vi "Setting.vi"() -> ()   [LabVIEW 2020]
uses:
  <userlib>/_MGI/1D Array/MGI Average/MGI Average (DBL[]).vi
  Global_Variable/Global.vi
  Libraries/S7/S7.lvlib
panel:
  in  "停止":bool
  in  "输入轴标定":bool
  out "标定曲线":cluster{dbl[], dbl[]}[](graph)
  # "配置标定"
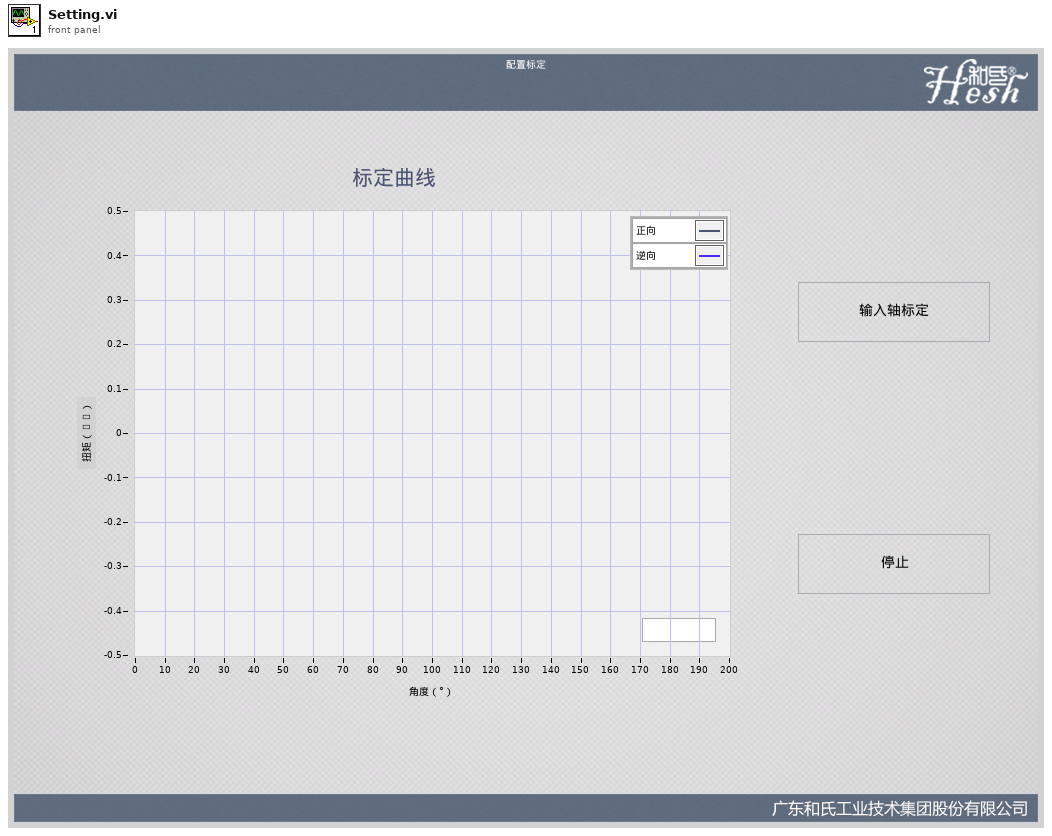
[diagram p1: front panel]
types:
  T1 = cluster{"输入旋转位移":sgl, "位移":sgl, "工装移载位移":sgl, "输入编码位移":sgl, "输入扭矩":sgl, "输出扭矩(小)":sgl, "拉压力":sgl, "吸收电流":sgl}
  T2 = cluster{"输入轴扭矩":dbl, "输出轴扭矩小量程":dbl, "输出轴扭矩大量程":dbl}
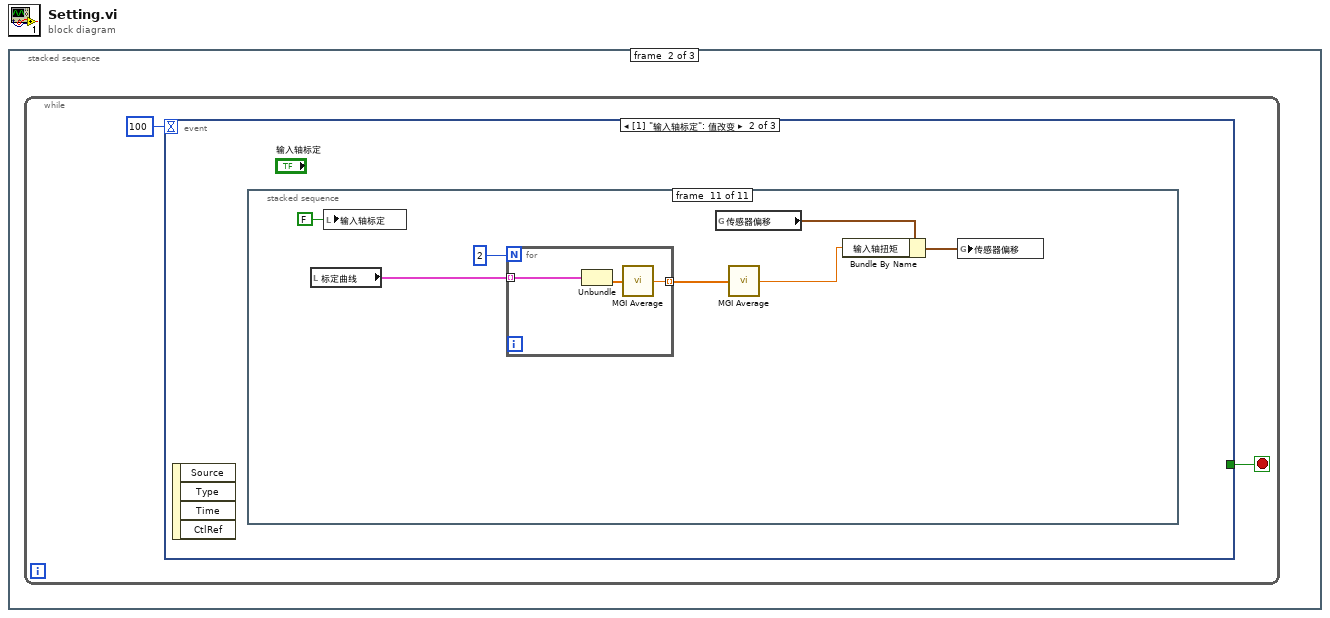
[diagram p0: block diagram]
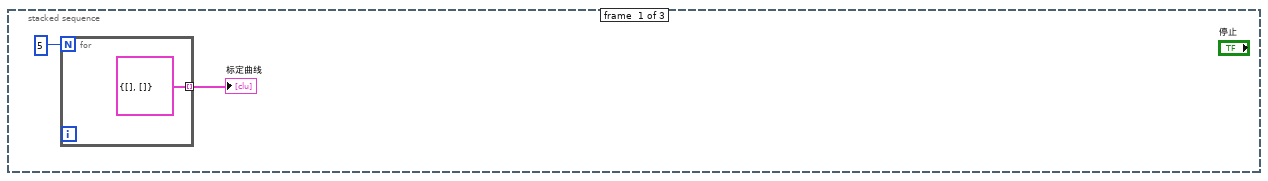
[diagram p2: hidden frame]
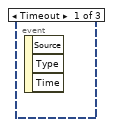
[diagram p3: hidden frame]
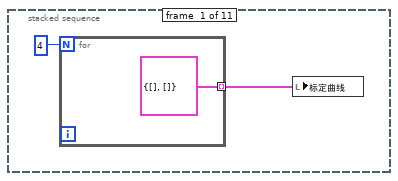
[diagram p4: hidden frame]
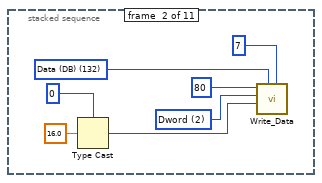
[diagram p5: hidden frame]
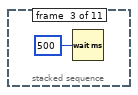
[diagram p6: hidden frame]
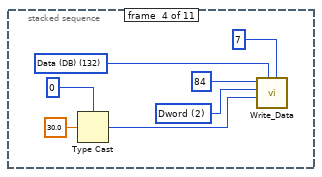
[diagram p7: hidden frame]
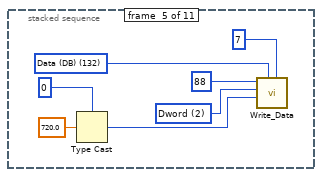
[diagram p8: hidden frame]
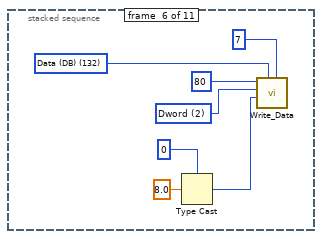
[diagram p9: hidden frame]
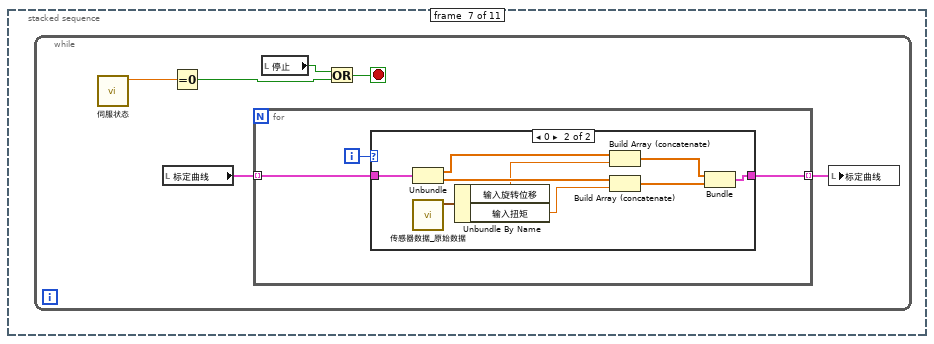
[diagram p10: hidden frame]
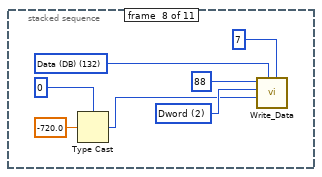
[diagram p12: hidden frame]
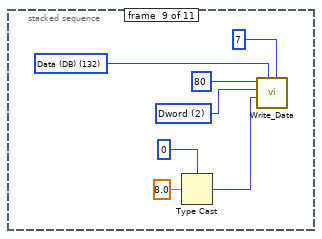
[diagram p13: hidden frame]
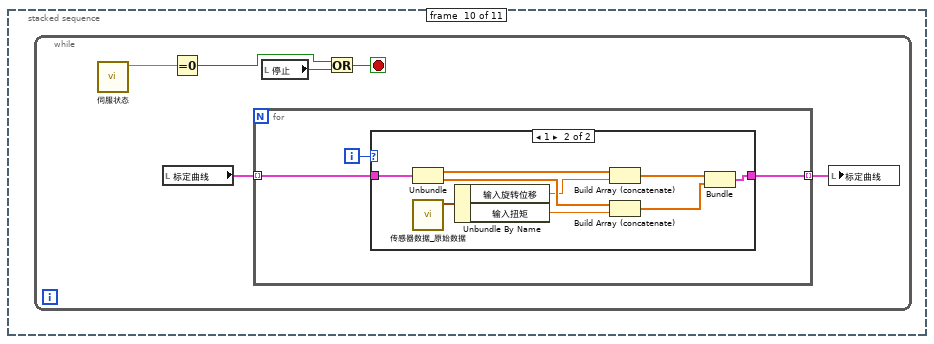
[diagram p14: hidden frame]
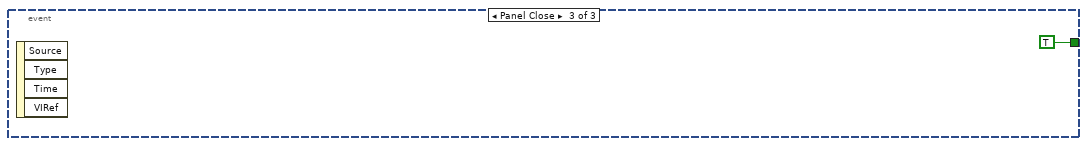
[diagram p16: hidden frame]
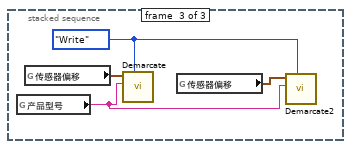
[diagram p17: hidden frame]
diagram:
  n1 = stacked-sequence {
    frame #0 {
      n2 = for {
        N: 5 -> [_]
        tunnel: [cluster{dbl[], dbl[]} {[], []}] -> w1 mode=indexing
      }
      "标定曲线" <- w1
    }
    frame #1 {
      n3 = while {
        stop <- w5 stop-if-true
        n4 = event shown="[1] \"输入轴标定\": 值改变" {
          selector: _ -> [_ _ _]
          dyn-events: _ -> [_ _ _]
          timeout: 100 -> [_ _ _]
          tunnel: [_ _ TRUE] -> w5
          event Timeout {
            n5 = event-data() -> ()  [unwired: 1 in, 3 out]
          }
          event "输入轴标定": Value Change {
            n6 = event-data() -> ()  [unwired: 1 in, 4 out]
            n7 = stacked-sequence {
              frame #0 {
                n8 = for {
                  N: 4 -> [_]
                  tunnel: [cluster{dbl[], dbl[]} {[], []}] -> w7 mode=indexing
                }
                n9 = local write "标定曲线"(w7) -> ()
              }
              frame #1 {
                w13 = u16 2 items=["byte", "word", "Dword"] ("数据类型")
                w15 = u8 132 items=["I/O (P)"=128, "Input (I)"=129, "Output (Q)"=130, "Bit Memory (M)"=131, "Data (DB)"=132, "Instance Data (DI)"=133, "Local Data (L)"=134, "Predecessor Local Data (VL)"=135] ("寄存器类型")
                n10 = Type Cast(type=u32 0, x=sgl 16.0 ("输入轴旋转绝对位置")) -> (*(type *) &x=w11:u32)
                n11 = call "Write_Data.vi"("DB #"=u16 7, "寄存器类型"=w15, "写入数据"=w11, "数据类型"=w13, "写入地址"=u32 80) -> ()  [unwired: 4 in, 3 out]
              }
              frame #2 {
                n12 = Wait (ms)(milliseconds to wait=u32 500 ("等待时间（毫秒）")) -> ()  [unwired: 1 out]
              }
              frame #3 {
                w21 = u16 2 items=["byte", "word", "Dword"] ("数据类型")
                w23 = u8 132 items=["I/O (P)"=128, "Input (I)"=129, "Output (Q)"=130, "Bit Memory (M)"=131, "Data (DB)"=132, "Instance Data (DI)"=133, "Local Data (L)"=134, "Predecessor Local Data (VL)"=135] ("寄存器类型")
                n13 = Type Cast(type=u32 0, x=sgl 30.0 ("输入轴旋转绝对位置")) -> (*(type *) &x=w19:u32)
                n14 = call "Write_Data.vi"("DB #"=u16 7, "寄存器类型"=w23, "写入数据"=w19, "数据类型"=w21, "写入地址"=u32 84) -> ()  [unwired: 4 in, 3 out]
              }
              frame #4 {
                w27 = u16 2 items=["byte", "word", "Dword"] ("数据类型")
                w28 = u8 132 items=["I/O (P)"=128, "Input (I)"=129, "Output (Q)"=130, "Bit Memory (M)"=131, "Data (DB)"=132, "Instance Data (DI)"=133, "Local Data (L)"=134, "Predecessor Local Data (VL)"=135] ("寄存器类型")
                n15 = Type Cast(type=u32 0, x=sgl 720.0 ("输入轴旋转绝对位置")) -> (*(type *) &x=w30:u32)
                n16 = call "Write_Data.vi"("DB #"=u16 7, "寄存器类型"=w28, "写入数据"=w30, "数据类型"=w27, "写入地址"=u32 88) -> ()  [unwired: 4 in, 3 out]
              }
              frame #5 {
                w34 = u16 2 items=["byte", "word", "Dword"] ("数据类型")
                w35 = u8 132 items=["I/O (P)"=128, "Input (I)"=129, "Output (Q)"=130, "Bit Memory (M)"=131, "Data (DB)"=132, "Instance Data (DI)"=133, "Local Data (L)"=134, "Predecessor Local Data (VL)"=135] ("寄存器类型")
                n17 = Type Cast(type=u32 0, x=sgl 8.0 ("输入轴旋转绝对位置")) -> (*(type *) &x=w37:u32)
                n18 = call "Write_Data.vi"("DB #"=u16 7, "寄存器类型"=w35, "写入数据"=w37, "数据类型"=w34, "写入地址"=u32 80) -> ()  [unwired: 4 in, 3 out]
              }
              frame #6 {
                n19 = while {
                  stop <- w42 stop-if-true
                  n20 = call "伺服状态.vi"() -> ("Status"=w39:sgl)  [unwired: 11 in]
                  n21 = local read "标定曲线"() -> (w41:cluster{dbl[], dbl[]}[])
                  n22 = Equal To 0?(x=w39) -> (x = 0?=w38:bool)
                  n23 = for {
                    tunnel: [w44] -> w40 mode=indexing
                    tunnel: w41 -> [w46] mode=indexing
                    i -> [w45]
                    n24 = case shown="0" w45 {
                      tunnel: [w47 w51] -> w44
                      tunnel: w46 -> [w47 w52]
                      frame Default {
                      }
                      frame 0 {
                        n25 = Unbundle(w52) -> (w56:dbl[], w55:dbl[])
                        n26 = call "传感器数据_原始数据.vi"() -> ("传感器读数"=w50:T1)  [unwired: 11 in]
                        n27 = Unbundle By Name(w50) -> ("输入旋转位移"=w49:sgl, "输入扭矩"=w48:sgl)
                        n28 = Build Array (concatenate)(w56, w49) -> (w54:dbl[])
                        n29 = Build Array (concatenate)(w55, w48) -> (w53:dbl[])
                        n30 = Bundle(w54, w53) -> (w51:cluster{dbl[], dbl[]})  [unwired: 1 in]
                      }
                    }
                  }
                  n31 = local read "停止"() -> (w43:bool)
                  n32 = Or(x=w43, y=w38) -> (x .or. y?=w42:bool)
                  n33 = local write "标定曲线"(w40) -> ()
                }
              }
              frame #7 {
                w61 = u16 2 items=["byte", "word", "Dword"] ("数据类型")
                w63 = u8 132 items=["I/O (P)"=128, "Input (I)"=129, "Output (Q)"=130, "Bit Memory (M)"=131, "Data (DB)"=132, "Instance Data (DI)"=133, "Local Data (L)"=134, "Predecessor Local Data (VL)"=135] ("寄存器类型")
                n34 = Type Cast(type=u32 0, x=sgl -720.0 ("输入轴旋转绝对位置")) -> (*(type *) &x=w59:u32)
                n35 = call "Write_Data.vi"("DB #"=u16 7, "寄存器类型"=w63, "写入数据"=w59, "数据类型"=w61, "写入地址"=u32 88) -> ()  [unwired: 4 in, 3 out]
              }
              frame #8 {
                w68 = u16 2 items=["byte", "word", "Dword"] ("数据类型")
                w70 = u8 132 items=["I/O (P)"=128, "Input (I)"=129, "Output (Q)"=130, "Bit Memory (M)"=131, "Data (DB)"=132, "Instance Data (DI)"=133, "Local Data (L)"=134, "Predecessor Local Data (VL)"=135] ("寄存器类型")
                n36 = Type Cast(type=u32 0, x=sgl 8.0 ("输入轴旋转绝对位置")) -> (*(type *) &x=w66:u32)
                n37 = call "Write_Data.vi"("DB #"=u16 7, "寄存器类型"=w70, "写入数据"=w66, "数据类型"=w68, "写入地址"=u32 80) -> ()  [unwired: 4 in, 3 out]
              }
              frame #9 {
                n38 = while {
                  stop <- w76 stop-if-true
                  n39 = call "伺服状态.vi"() -> ("Status"=w72:sgl)  [unwired: 11 in]
                  n40 = local read "标定曲线"() -> (w74:cluster{dbl[], dbl[]}[])
                  n41 = Equal To 0?(x=w72) -> (x = 0?=w71:bool)
                  n42 = for {
                    tunnel: [w77] -> w73 mode=indexing
                    tunnel: w74 -> [w79] mode=indexing
                    i -> [w78]
                    n43 = case shown="1" w78 {
                      tunnel: [w80 w84] -> w77
                      tunnel: w79 -> [w80 w85]
                      frame Default {
                      }
                      frame 1 {
                        n44 = Unbundle(w85) -> (w89:dbl[], w88:dbl[])
                        n45 = call "传感器数据_原始数据.vi"() -> ("传感器读数"=w83:T1)  [unwired: 11 in]
                        n46 = Unbundle By Name(w83) -> ("输入旋转位移"=w81:sgl, "输入扭矩"=w82:sgl)
                        n47 = Build Array (concatenate)(w89, w81) -> (w87:dbl[])
                        n48 = Build Array (concatenate)(w88, w82) -> (w86:dbl[])
                        n49 = Bundle(w87, w86) -> (w84:cluster{dbl[], dbl[]})  [unwired: 1 in]
                      }
                    }
                  }
                  n50 = local read "停止"() -> (w75:bool)
                  n51 = Or(x=w71, y=w75) -> (x .or. y?=w76:bool)
                  n52 = local write "标定曲线"(w73) -> ()
                }
              }
              frame #10 {
                n53 = local read "标定曲线"() -> (w90:cluster{dbl[], dbl[]}[])
                n54 = local write "输入轴标定"(FALSE ("输入轴标定")) -> ()
                n55 = for {
                  N: 2 -> [_]
                  tunnel: w90 -> [w99] mode=indexing
                  tunnel: [w97] -> w91 mode=indexing
                  n56 = Unbundle(w99) -> (w98:dbl[])  [unwired: 1 out]
                  n57 = call-poly <userlib>:"MGI Average.vi"("Double[]"=w98) -> ("Average"=w97:dbl)  [unwired: 1 in]
                }
                n58 = global read "传感器偏移.vi" "传感器偏移"() -> (w93:T2)
                n59 = call-poly <userlib>:"MGI Average.vi"("Double[]"=w91) -> ("Average"=w95:dbl)  [unwired: 1 in]
                n60 = Bundle By Name(cluster=w93, "输入轴扭矩"=w95) -> (w94:T2)
                n61 = global write "传感器偏移.vi" "传感器偏移"(w94) -> ()
              }
            }
          }
          event Panel Close {
            n62 = event-data() -> ()  [unwired: 1 in, 4 out]
          }
        }
      }
    }
    frame #2 {
      w103 = enum16{"Read", "Write"}."Write" ("Mode")
      n63 = global read "Global.vi" "产品型号"() -> (w101:string)
      n64 = global read "传感器偏移.vi" "传感器偏移"() -> (w104:T2)
      n65 = call "Demarcate.vi"("Mode"=w103, "Section"=w101, "Sensor IN"=w104) -> ()  [unwired: 7 in, 2 out]
      n66 = global read "传感器偏移.vi" "传感器偏移"() -> (w102:T2)
      n67 = call "Demarcate2.vi"("Mode"=w103, "Section"=w101, "Sensor IN"=w102) -> ()  [unwired: 7 in, 2 out]
    }
  }
